vi "Press And Hold Button .vi"(0 "GEA2 Reference In":refnum<k24>, 1 "Delay Time (s)":dbl=3.25 format="%#_13g", 5 "Standalone?":bool, 7 "Button":T2=enum."SW201 - My Cycle", 9 "GEA Inputs":T1 {"Destination" format="%.0x"; "Source" format="%.0x"}, 11 "Error In":errorcluster) -> (4 "GEA2 Reference Out":refnum<k24>, 15 "Error Out":errorcluster)   [LabVIEW 2016, in "2015 VA Washer.lvlib"]
uses:
  Projects/2015 VA Washer.lvlib
  type defs/UI Buttons.ctl
  C:/Automation/DLLs/PC Dot Net/GeaCommunication.dll
  Common/LabVIEW GEA2 Toolkit/LabVIEW_GEA2_Toolkit.lvlibp/type defs/Source_Destination.ctl
  Common/LabVIEW GEA2 Toolkit/LabVIEW_GEA2_Toolkit.lvlibp/type defs/ERD Write Data In.ctl
  Common/LabVIEW GEA2 Toolkit/LabVIEW_GEA2_Toolkit.lvlibp/type defs/Data Type.ctl
  Common/LabVIEW GEA2 Toolkit/LabVIEW_GEA2_Toolkit.lvlibp
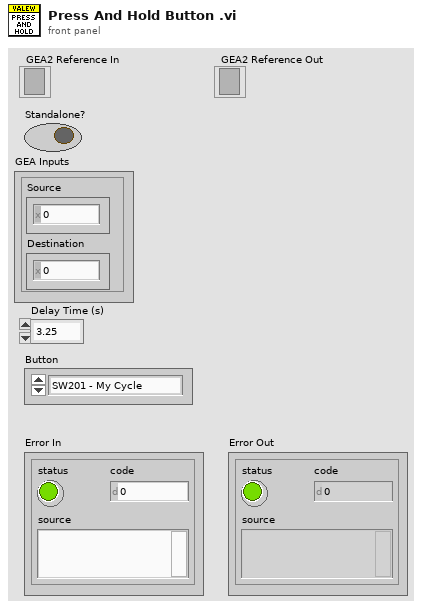
[diagram p1: front panel]
types:
  T1 = typedef "LabVIEW_GEA2_Toolkit.lvlibp/Source_Destination.ctl" = cluster{"Source":u8, "Destination":u8}
  T2 = typedef "2015 VA Washer.lvlib/UI Buttons.ctl" = enum16{"Switch Off", "SW201 - My Cycle", "SW202 - Delay Wash", "SW203 - Extra Rinse", "SW204 - Signal / Volume", "SW205 - Spin", "SW206 - Deep Rinse / Fab Soft", "SW207 - Soil", "SW208 - Auto Soak", "SW209 - Temp", "SW210 - Warm Rinse", "SW211 - Deep Fill", "SW212 - Stain Remover", "SW213 - Power", "SW222 - Control Lock", "SW214 - Start / Pause", "SW301 - Start/Pause LE", "SW302 - Option Button LE"}
  T3 = typedef "LabVIEW_GEA2_Toolkit.lvlibp/ERD Write Data In.ctl" = cluster{"ERD Number":u16, "Data Type":T4, "Data":string}
  T4 = typedef "LabVIEW_GEA2_Toolkit.lvlibp/Data Type.ctl" = enum16{"string", "boolean", "uint8_t", "uint16_t", "uint32_t", "uint64_t", "int8_t", "int16_t", "int32_t", "int64_t"}
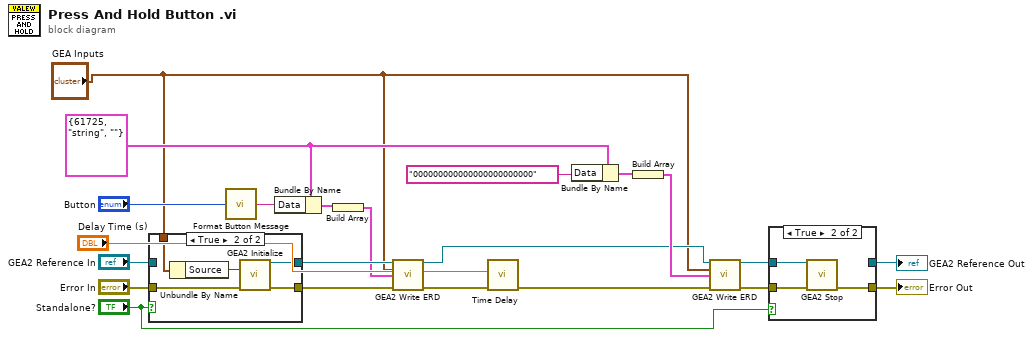
[diagram p0: block diagram]
diagram:
  w2 = T3 {"ERD Number"=61725, "Data Type"=enum."string", "Data"=""} ("ERD Write Data In")
  n1 = case shown="True" "Standalone?" {
    tunnel: "Error In" -> [w23 w29]
    tunnel: [w23 w28] -> w15
    tunnel: "GEA2 Reference In" -> [w24 _]
    tunnel: [w24 w27] -> w13
    tunnel: "GEA Inputs" -> [_ w25]
    frame False {
    }
    frame True {
      n2 = Unbundle By Name(w25) -> ("Source"=w26:u8)
      n3 = call "GEA2 Initialize.vi"("Source Address"=w26, "error in"=w29) -> ("GEA2 Reference Out"=w27:refnum<k24>, "error out"=w28:errorcluster)  [unwired: 11 in, 1 out]
    }
  }
  n4 = call "Format Button Message.vi"("Switch"="Button") -> ("Switch Message"=w12:string)  [unwired: 14 in]
  n5 = Bundle By Name(cluster=w2, "Data"=w12) -> (w11:T3)
  n6 = Build Array(w11) -> (w10:T3[])
  n7 = call "GEA2 Write ERD.vi"("GEA2 Reference In"=w13, "GEA Inputs"="GEA Inputs", "Write ERD List"=w10, "Error In"=w15) -> ("GEA2 Reference Out"=w3:refnum<k24>, "Error Out"=w14:errorcluster)  [unwired: 9 in, 1 out]
  n8 = call "Time Delay"("error in (no error)"=w14, "Delay Time (s)"="Delay Time (s)") -> ("error out"=w8:errorcluster)  [unwired: 9 in]
  n9 = Bundle By Name(cluster=w2, "Data"="000000000000000000000000" ("Message")) -> (w5:T3)
  n10 = Build Array(w5) -> (w4:T3[])
  n11 = call "GEA2 Write ERD.vi"("GEA2 Reference In"=w3, "GEA Inputs"="GEA Inputs", "Write ERD List"=w4, "Error In"=w8) -> ("GEA2 Reference Out"=w9:refnum<k24>, "Error Out"=w7:errorcluster)  [unwired: 9 in, 1 out]
  n12 = case shown="True" "Standalone?" {
    tunnel: [w30 w34] -> w18
    tunnel: w9 -> [w31 w33]
    tunnel: [w31 _] -> w17
    tunnel: w7 -> [w30 w32]
    frame False {
    }
    frame True {
      n13 = call "GEA2 Stop.vi"("GEA2 Reference In"=w33, "Error In"=w32) -> ("Error Out"=w34:errorcluster)  [unwired: 13 in]
    }
  }
  "Error Out" <- w18
  "GEA2 Reference Out" <- w17
